vi "Unlock Publication.vi"(6 "Publisher ID":string, 8 "error in (no error)":errorcluster, 9 "Datum Type":variant, 10 "Datum Name":string, 11 "Mediator In":refnum<class "Mediator.lvclass">) -> (0 "error out":errorcluster, 3 "Mediator Out":refnum<class "Mediator.lvclass">)   [LabVIEW 2015, in "Mediator.lvlib" / "Mediator.lvclass"]
doc: "<License>\nCopyright © 2017 Composed Systems, LLC | All rights reserved\nwww.composed.io\n\nAuthor: Ethan Stern <ethan.stern@composed.io>\n\nThis software is provided \"AS IS\" WITHOUT WARRANTIES, either express or implied, AND IS FOR EDUCATIONAL PURPOSES ONLY.\n</License>"
uses:
  Mediator.lvclass
  Mediator.lvclass/Mediator.ctl
  Topic Messages/Unlock Topic Msg/Unlock Topic Msg.lvclass/Unlock Topic Msg.ctl
  <vilib>/ActorFramework/Message Enqueuer/Message Enqueuer.lvclass/Message Enqueuer.ctl
  <vilib>/ActorFramework/Message Enqueuer/Enqueue.vi
  <vilib>/ActorFramework/Message Priority Queue/Priority Enqueue.vi
  Topic Messages/Unlock Topic Msg/Unlock Topic Msg.lvclass
  TopicLookupTable/TopicLookupTable.lvclass
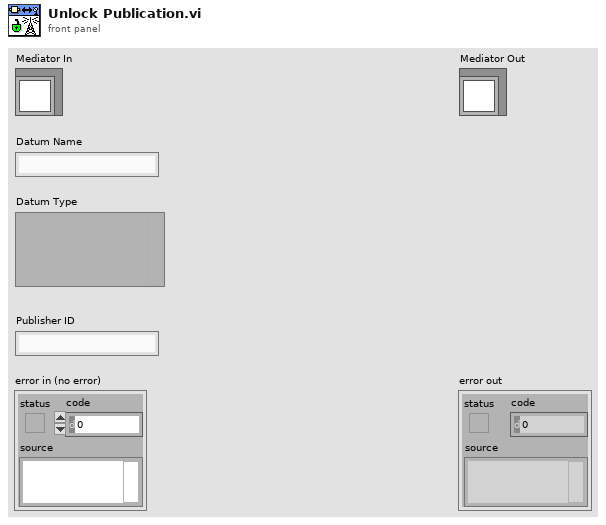
[diagram p1: front panel]
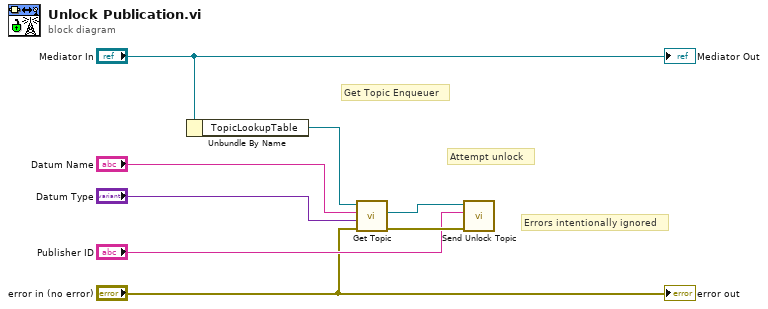
[diagram p0: block diagram]
diagram:
  # "Errors intentionally ignored"
  # "Attempt unlock"
  # "Get Topic Enqueuer"
  n1 = Unbundle By Name("Mediator In") -> ("TopicLookupTable"=w7:refnum<data-value>)
  n2 = call "Get Topic.vi"("error in (no error)"="error in (no error)", "Topic Type"="Datum Type", "Topic Name"="Datum Name", "TopicLookupTable"=w7) -> ("error out"=w3:errorcluster, "Topic Enqueuer"=w4:refnum<class "Message Enqueuer.lvclass">)  [unwired: 5 in, 1 out]
  n3 = call "Send Unlock Topic.vi"("error in (no error)"=w3, "Publisher ID"="Publisher ID", "Message Enqueuer"=w4) -> ()  [unwired: 7 in, 2 out]
  "error out" <- "error in (no error)"
  "Mediator Out" <- "Mediator In"
